vi "acquisitionReorderFrames.vi"(1 "flip z":bool, 2 "reference z":dbl[](array[numeric]), 3 "current z":dbl[](array[numeric]), 4 "frames in":u16[][][](array[numeric])) -> (0 "frames out":u16[][][](array[numeric]))   [LabVIEW 2017]
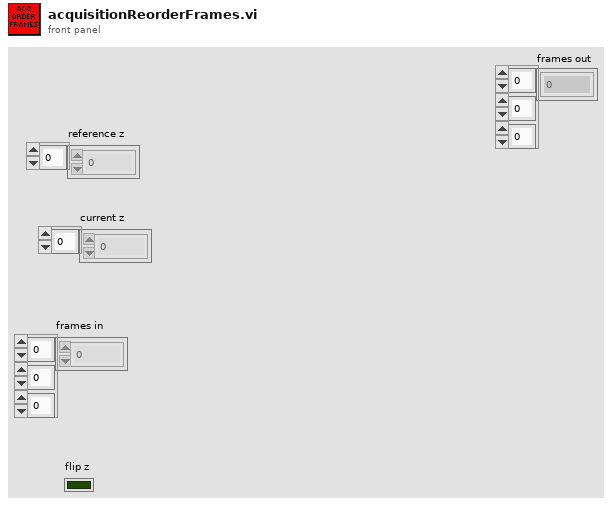
[diagram p1: front panel]
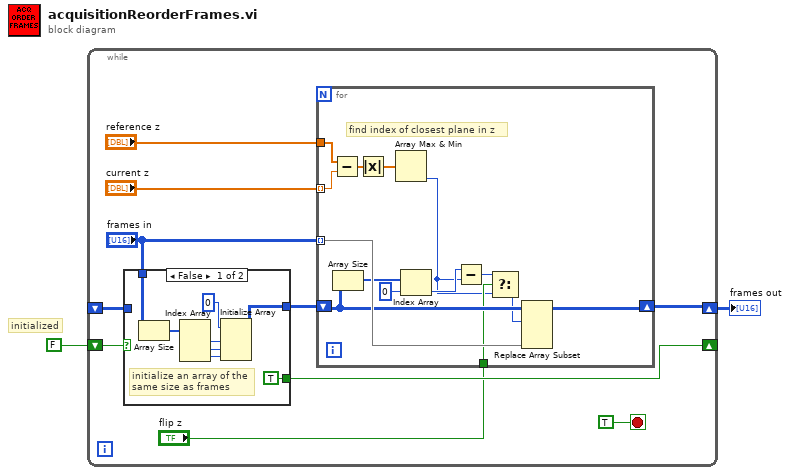
[diagram p0: block diagram]
diagram:
  # "initialized"
  n1 = while {
    shift-right: [w6] -> w1
    shift-left: _ -> [w8]
    shift-right: [w5] -> _
    shift-left: FALSE -> [w10]
    stop <- TRUE stop-if-true
    n2 = case shown="False" w10 {
      selector: w10 -> [_ w21]
      tunnel: "frames in" -> [w20 _]
      tunnel: [w18 w22] -> w7
      tunnel: w8 -> [_ w22]
      tunnel: [TRUE w21] -> w5
      frame False {
        # "initialize an array of the\nsame size as frames"
        n3 = Array Size(array=w20) -> (size(s)=w17:i32[])
        n4 = Index Array(array=w17) -> (element #1=w16:i32, element #2=w15:i32, element #3=w14:i32)  [unwired: 3 in]
        n5 = Initialize Array(u16 0 ("element"), w16, w15, w14) -> (w18:u16[][][])
      }
      frame True {
      }
    }
    n6 = for {
      tunnel: "current z" -> [w35] mode=indexing
      tunnel: "reference z" -> [w36]
      tunnel: "frames in" -> [w32] mode=indexing
      shift-right: [w31] -> w6
      shift-left: w7 -> [w30]
      tunnel: "flip z" -> [w27]
      # "find index of closest plane in z"
      n7 = Subtract(x=w36, y=w35) -> (x-y=w34:dbl[])
      n8 = Array Size(array=w30) -> (size(s)=w29:i32[])
      n9 = Absolute Value(x=w34) -> (abs(x)=w33:dbl[])
      n10 = Array Max & Min(array=w33) -> (min index (indices)=w24:i32)  [unwired: 3 out]
      n11 = Index Array(array=w29, index=0) -> (element=w25:i32)
      n12 = Subtract(x=w25, y=w24) -> (x-y=w26:i32)
      n13 = Select(t=w26, s=w27, f=w24) -> (s? t:f=w23:i32)
      n14 = Replace Array Subset(array=w30, new element=w32, index (dim 0)=w23) -> (w31:u16[][][])  [unwired: 2 in]
    }
  }
  "frames out" <- w1
